vi "generate_staircase_waveform.vi"(0 "Start (µm)":dbl, 1 "Sweep Time":u32, 2 "Left Padding":u32, 3 "Right Padding":u32, 5 "End (µm)":dbl, 7 "Step Size (µm)":dbl, 9 "Number Slices":u32, 11 "Sweep Interval":u32) -> (8 "array":dbl[](array[numeric]))   [LabVIEW 2013]
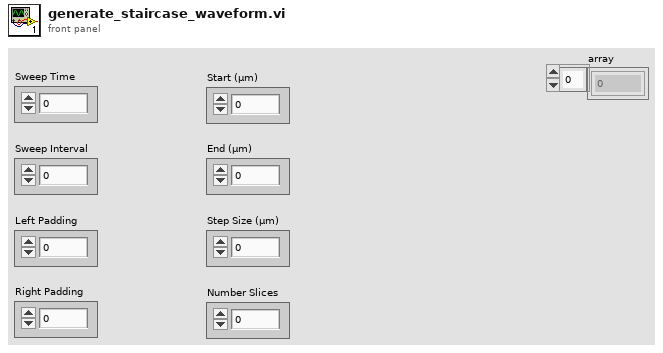
[diagram p1: front panel]
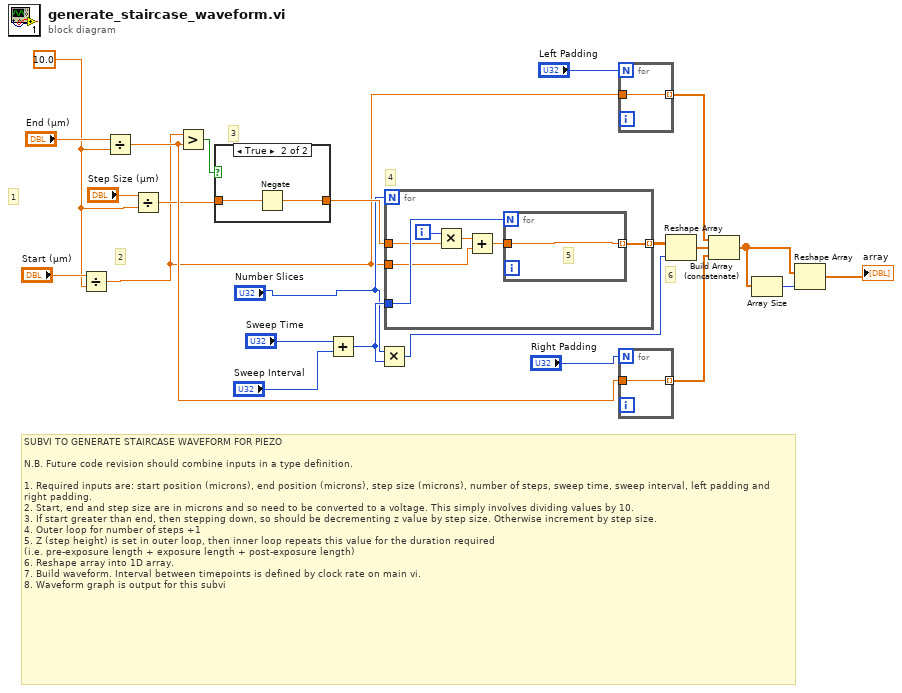
[diagram p0: block diagram]
diagram:
  w1 = 10.0 ("y")
  # "6"
  # "4"
  # "3"
  # "2"
  # "1"
  # "SUBVI TO GENERATE STAIRCASE WAVEFORM FOR PIEZO\n\nN.B. Future code revision should combine inputs in a type definition.\n\n1. Required inputs are: start position (microns), end position (microns), step size (microns), number of steps, sweep time, sweep interval, left padding and right padding.\n2. Start, end and step size are in microns and so need to be converted to a voltage. This simply involves dividing values by 10.\n3. If start greater than end, then stepping down, so should be decrementing z value by step size. Otherwise increment by step size. \n4. Outer loop for number of steps +1 \n5. Z (step height) is set in outer loop, then inner loop repeats this value for the duration required \n(i.e. pre-exposure length + exposure length + post-exposure length)\n6. Reshape array into 1D array.\n7. Build waveform. Interval between timepoints is defined by clock rate on main vi.\n8. Waveform graph is output for this subvi"
  n1 = Divide(x="Start (µm)", y=w1) -> (x/y=w3:dbl)
  n2 = Divide(x="End (µm)", y=w1) -> (x/y=w7:dbl)
  n3 = Divide(x="Step Size (µm)", y=w1) -> (x/y=w5:dbl)
  n4 = Greater?(x=w3, y=w7) -> (0:w23:bool)
  n5 = case shown="True" w23 {
    tunnel: w5 -> [w24 w26]
    tunnel: [w24 w25] -> w22
    frame False {
    }
    frame True {
      n6 = Negate(x=w26) -> (-x=w25:dbl)
    }
  }
  n7 = Add(x="Sweep Time", y="Sweep Interval") -> (x+y=w19:u32)
  n8 = Multiply(x="Number Slices", y=w19) -> (x*y=w20:u32)
  n9 = for {
    N: "Number Slices" -> [_]
    tunnel: w19 -> [w33]
    tunnel: w22 -> [w32]
    tunnel: w3 -> [w29]
    tunnel: [w28] -> w21 mode=indexing
    i -> [w27]
    n10 = Multiply(x=w27, y=w32) -> (x*y=w31:dbl)
    n11 = Add(x=w31, y=w29) -> (x+y=w30:dbl)
    n12 = for {
      N: w33 -> [_]
      tunnel: w30 -> [w34]
      tunnel: [w34] -> w28 mode=indexing
      # "5"
    }
  }
  n13 = for {
    N: "Left Padding" -> [_]
    tunnel: w3 -> [w35]
    tunnel: [w35] -> w14 mode=indexing
  }
  n14 = for {
    N: "Right Padding" -> [_]
    tunnel: w7 -> [w36]
    tunnel: [w36] -> w12 mode=indexing
  }
  n15 = Reshape Array(w21, w20) -> (w13:dbl[])
  n16 = Build Array (concatenate)(w14, w13, w12) -> (w11:dbl[])
  n17 = Array Size(array=w11) -> (size(s)=w10:i32)
  n18 = Reshape Array(w11, w10) -> (→"array":dbl[])
